vi "test_orientation_tester.vi"() -> ()   [LabVIEW 2026]
uses:
  <vilib>/Utility/error.llb/Trim Whitespace One-Sided.vi
panel:
  out "error out 2":errorcluster
  out "String":string
  out "error out":errorcluster
  in  "Serial Port":refnum<visa-resource-name>="N/A"
  in  "stop":bool
  in  "Tab Control":enum32{"Integrated Circuit Testing"}(tab)
  out "Orientation OK":bool
  out "Detected IC":string
  out "Current":dbl(graph)
  in  "IC Select":u16(ring) items=["7408", "7432", "7404"]
  out "D1":bool
  out "D2":bool
  out "D3":bool
  out "D4":bool
  out "D5":bool
  out "D6":bool
  out "D8":bool
  out "D9":bool
  out "D10":bool
  out "D11":bool
  out "D12":bool
  out "D13":bool
  in  "Start Test":bool
  out "Tests Ran":dbl
  out "PASS":bool
  out "FAIL":bool
  out "Passed":dbl
  out "Failed":dbl
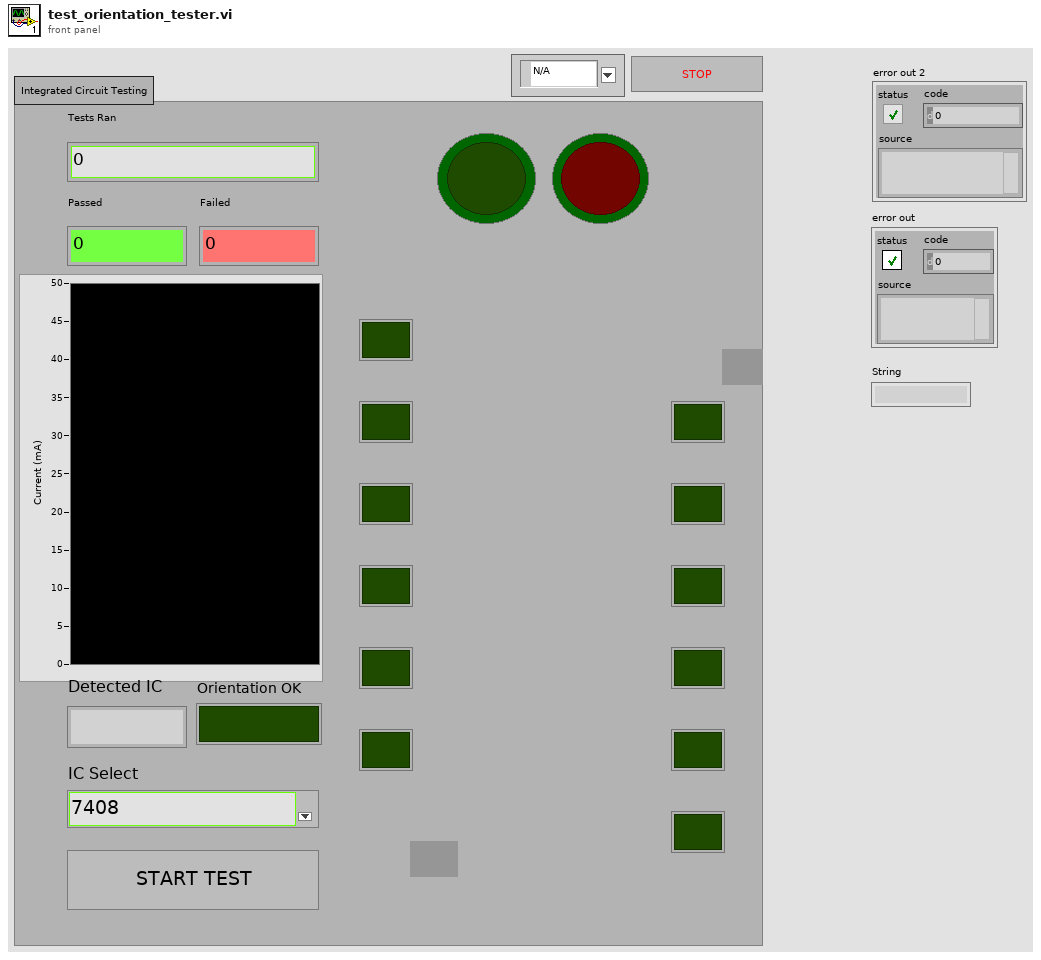
[diagram p1: front panel]
types:
  T1 = enum16{"Standard", "Buffered", "CRLF", "Immediate"}
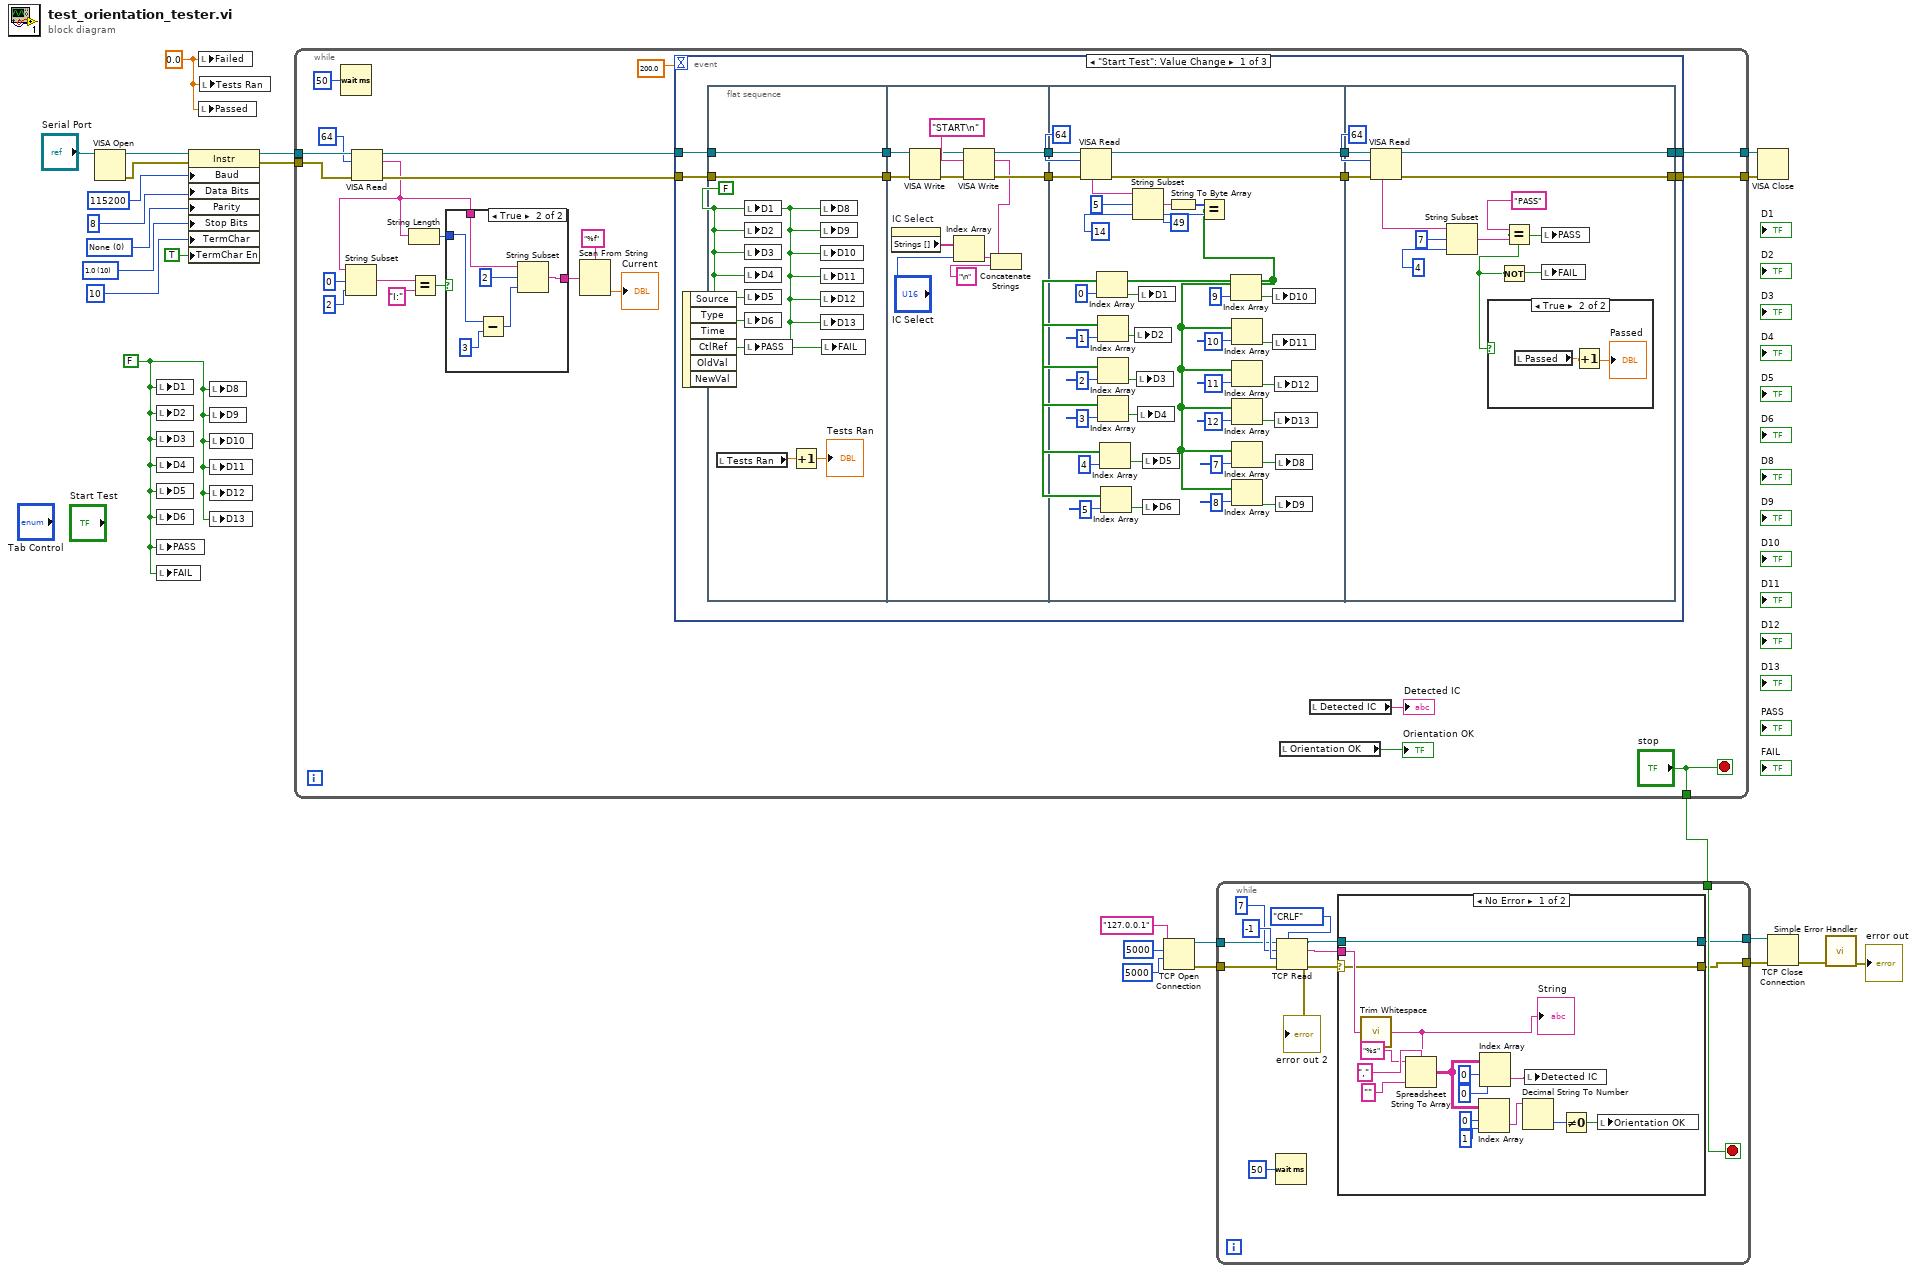
[diagram p0: block diagram]
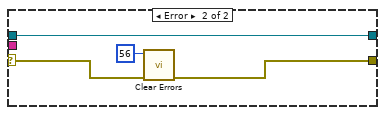
[diagram p2: hidden frame]
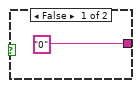
[diagram p3: hidden frame]
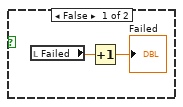
[diagram p4: hidden frame]
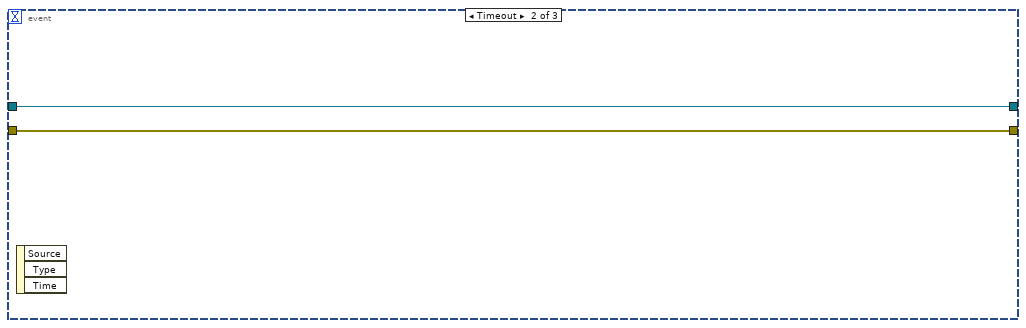
[diagram p5: hidden frame]
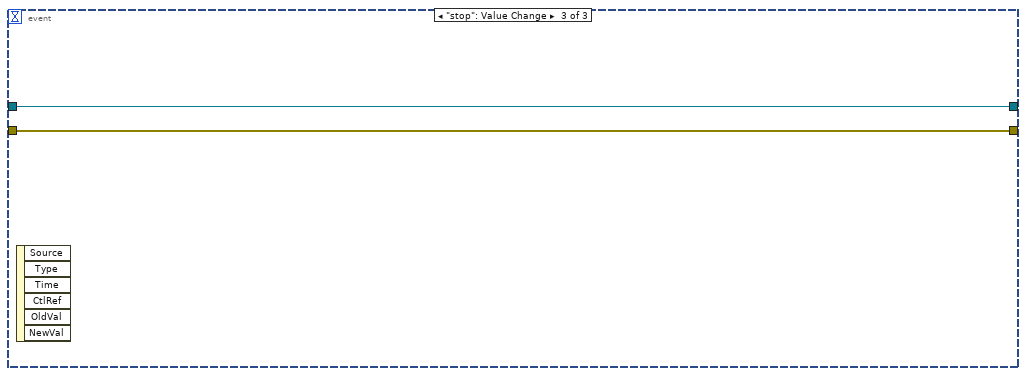
[diagram p6: hidden frame]
diagram:
  w8 = 0.0 ("Failed")
  w12 = FALSE ("D1")
  w17 = u16 10 items=["1.0"=10, "1.5"=15, "2.0"=20] ("Serial Settings:Stop Bits")
  w18 = u16 0 items=["None", "Odd", "Even", "Mark", "Space"] ("Serial Settings:Parity")
  n1 = VISA Open(VISA resource name="Serial Port") -> (VISA resource name=w24:refnum<visa-resource-name>, error out=w22:errorcluster)  [unwired: 4 in]
  n2 = local write "D1"(w12) -> ()
  n3 = local write "D2"(w12) -> ()
  n4 = local write "D3"(w12) -> ()
  n5 = local write "D4"(w12) -> ()
  n6 = local write "D5"(w12) -> ()
  n7 = local write "D6"(w12) -> ()
  n8 = local write "PASS"(w12) -> ()
  n9 = local write "FAIL"(w12) -> ()
  n10 = property class="Instr"(reference=w24, error in=w22, "Baud"=u32 115200 ("Serial Settings:Baud Rate"), "Data Bits"=u16 8 ("Serial Settings:Data Bits"), "Parity"=w18, "Stop Bits"=w17, "TermChar"=u8 10 ("Message Based Settings:Termination Character"), "TermChar En"=TRUE ("Message Based Settings:Termination Character Enable")) -> (reference out=w23:refnum<visa-resource-name>, error out=w21:errorcluster)
  n11 = local write "Failed"(w8) -> ()
  n12 = local write "Passed"(w8) -> ()
  n13 = local write "Tests Ran"(w8) -> ()
  n14 = local write "D8"(w12) -> ()
  n15 = local write "D9"(w12) -> ()
  n16 = local write "D10"(w12) -> ()
  n17 = local write "D11"(w12) -> ()
  n18 = local write "D12"(w12) -> ()
  n19 = local write "D13"(w12) -> ()
  n20 = while {
    tunnel: w23 -> [w47]
    tunnel: w21 -> [w45]
    tunnel: [w42] -> w14
    tunnel: [w41] -> w13
    tunnel: ["stop"] -> w6
    stop <- "stop" stop-if-true
    n21 = Wait (ms)(milliseconds to wait=u32 50) -> ()  [unwired: 1 out]
    n22 = VISA Read(VISA resource name=w47, byte count=u32 64, error in (no error)=w45) -> (VISA resource name out=w44:refnum<visa-resource-name>, read buffer=w35:string, error out=w43:errorcluster)  [unwired: 1 out]
    n23 = String Subset(string=w35, offset (0)=0, length (rest)=2 ("length (rest)")) -> (substring=w34:string)
    n24 = String Length(string=w35) -> (length=w36:i32)
    n25 = Equal?(x=w34, y="I:") -> (x = y?=w33:bool)
    n26 = case shown="True" w33 {
      tunnel: w36 -> [_ w53]
      tunnel: ["0" w50] -> w31
      tunnel: w35 -> [_ w49]
      frame False {
      }
      frame True {
        n27 = Subtract(x=w53, y=3) -> (x-y=w51:i32)
        n28 = String Subset(string=w49, offset (0)=2, length (rest)=w51) -> (substring=w50:string)
      }
    }
    n29 = Scan From String(format string="%f", input string=w31) -> (output 1=→"Current":dbl)  [unwired: 3 in, 3 out]
    n30 = event shown="[0] \"Start Test\": Value Change" {
      selector: _ -> [_ _ _]
      dyn-events: _ -> [_ _ _]
      timeout: 200.0 -> [_ _ _]
      tunnel: w44 -> [w63 w135 w137]
      tunnel: w43 -> [w61 w134 w136]
      tunnel: [w60 w135 w137] -> w42
      tunnel: [w59 w134 w136] -> w41
      event "Start Test": Value Change {
        n31 = event-data() -> ()  [unwired: 1 in, 6 out]
        n32 = flat-sequence {
          tunnel: [w69] -> w64
          tunnel: w63 -> [w69]
          tunnel: [w68] -> w62
          tunnel: w61 -> [w68]
          tunnel: w64 -> [w78]
          tunnel: w62 -> [w76]
          tunnel: [w81] -> w58
          tunnel: [w80] -> w57
          tunnel: w58 -> [w116]
          tunnel: w57 -> [w117]
          tunnel: [w115] -> w56
          tunnel: [w114] -> w55
          tunnel: [w126] -> w59
          tunnel: [w127] -> w60
          tunnel: w56 -> [w129]
          tunnel: w55 -> [w128]
          frame #0 {
            w67 = FALSE ("D1")
            n33 = local read "Tests Ran"() -> (w66:dbl)
            n34 = local write "D1"(w67) -> ()
            n35 = local write "D2"(w67) -> ()
            n36 = local write "D3"(w67) -> ()
            n37 = local write "D4"(w67) -> ()
            n38 = local write "D5"(w67) -> ()
            n39 = local write "D6"(w67) -> ()
            n40 = local write "PASS"(w67) -> ()
            n41 = Increment(x=w66) -> (x+1=→"Tests Ran":dbl)
            n42 = local write "D8"(w67) -> ()
            n43 = local write "D9"(w67) -> ()
            n44 = local write "D10"(w67) -> ()
            n45 = local write "D11"(w67) -> ()
            n46 = local write "D12"(w67) -> ()
            n47 = local write "D13"(w67) -> ()
            n48 = local write "FAIL"(w67) -> ()
          }
          frame #1 {
            n49 = property on="IC Select" class="Ring (strict)"() -> ("Strings []"=w74:string[])  [unwired: 2 in, 2 out]
            n50 = Index Array(array=w74, index="IC Select") -> (element=w72:string)
            n51 = Concatenate Strings(w72, "\n" ("string")) -> (w70:string)
            n52 = VISA Write(VISA resource name=w78, write buffer=w70, error in (no error)=w76) -> (VISA resource name out=w77:refnum<visa-resource-name>, error out=w75:errorcluster)  [unwired: 1 out]
            n53 = VISA Write(VISA resource name=w77, write buffer="START\n", error in (no error)=w75) -> (VISA resource name out=w81:refnum<visa-resource-name>, error out=w80:errorcluster)  [unwired: 1 out]
          }
          frame #2 {
            n54 = VISA Read(VISA resource name=w116, byte count=u32 64, error in (no error)=w117) -> (VISA resource name out=w115:refnum<visa-resource-name>, read buffer=w108:string, error out=w114:errorcluster)  [unwired: 1 out]
            n55 = String Subset(string=w108, offset (0)=5, length (rest)=14 ("length (rest)")) -> (substring=w112:string)
            n56 = String To Byte Array(string=w112) -> (unsigned byte array=w111:u8[])
            n57 = Equal?(x=w111, y=u8 49) -> (x = y?=w83:bool[])
            n58 = Index Array(array=w83, index=0) -> (element=w107:bool)
            n59 = Index Array(array=w83, index=1) -> (element=w103:bool)
            n60 = Index Array(array=w83, index=2) -> (element=w102:bool)
            n61 = Index Array(array=w83, index=3) -> (element=w105:bool)
            n62 = Index Array(array=w83, index=4) -> (element=w106:bool)
            n63 = Index Array(array=w83, index=5) -> (element=w104:bool)
            n64 = local write "D2"(w103) -> ()
            n65 = local write "D3"(w102) -> ()
            n66 = local write "D4"(w105) -> ()
            n67 = local write "D1"(w107) -> ()
            n68 = local write "D5"(w106) -> ()
            n69 = local write "D6"(w104) -> ()
            n70 = Index Array(array=w83, index=9) -> (element=w93:bool)
            n71 = Index Array(array=w83, index=10) -> (element=w92:bool)
            n72 = Index Array(array=w83, index=11) -> (element=w91:bool)
            n73 = Index Array(array=w83, index=12) -> (element=w90:bool)
            n74 = Index Array(array=w83, index=7) -> (element=w95:bool)
            n75 = Index Array(array=w83, index=8) -> (element=w94:bool)
            n76 = local write "D10"(w93) -> ()
            n77 = local write "D11"(w92) -> ()
            n78 = local write "D12"(w91) -> ()
            n79 = local write "D13"(w90) -> ()
            n80 = local write "D8"(w95) -> ()
            n81 = local write "D9"(w94) -> ()
          }
          frame #3 {
            n82 = VISA Read(VISA resource name=w129, byte count=u32 64, error in (no error)=w128) -> (VISA resource name out=w127:refnum<visa-resource-name>, read buffer=w122:string, error out=w126:errorcluster)  [unwired: 1 out]
            n83 = String Subset(string=w122, offset (0)=7, length (rest)=4 ("length (rest)")) -> (substring=w118:string)
            n84 = Equal?(x="PASS", y=w118) -> (x = y?=w119:bool)
            n85 = case shown="True" w119 {
              frame False {
                n86 = local read "Failed"() -> (w130:dbl)
                n87 = Increment(x=w130) -> (x+1=→"Failed":dbl)
              }
              frame True {
                n88 = local read "Passed"() -> (w132:dbl)
                n89 = Increment(x=w132) -> (x+1=→"Passed":dbl)
              }
            }
            n90 = Not(x=w119) -> (.not. x?=w121:bool)
            n91 = local write "PASS"(w119) -> ()
            n92 = local write "FAIL"(w121) -> ()
          }
        }
      }
      event Timeout {
        n93 = event-data() -> ()  [unwired: 1 in, 3 out]
      }
      event "stop": Value Change {
        n94 = event-data() -> ()  [unwired: 1 in, 6 out]
      }
    }
    n95 = local read "Orientation OK"() -> (→"Orientation OK":bool)
    n96 = local read "Detected IC"() -> (→"Detected IC":string)
  }
  n97 = TCP Open Connection(address="127.0.0.1", remote port or service name=u16 5000, timeout ms (60000)=5000) -> (connection ID=w7:refnum<k5>, error out=w4:errorcluster)  [unwired: 2 in]
  n98 = while {
    tunnel: w7 -> [w146]
    tunnel: w6 -> [w145]
    tunnel: [w143] -> w5
    tunnel: w4 -> [w144]
    tunnel: [w140] -> w2
    stop <- w145 stop-if-true
    n99 = Wait (ms)(milliseconds to wait=u32 50) -> ()  [unwired: 1 out]
    n100 = TCP Read(connection ID=w146, bytes to read=7, error in (no error)=w144, 7:T1."CRLF" ("mode (standard)"), 9:-1 ("timeout ms (25000)")) -> (connection ID out=w142:refnum<k5>, data out=w141:string, error out=w138:errorcluster)
    "error out 2" <- w138
    n101 = case shown="No Error" w138 {
      selector: w138 -> [w153 w168]
      tunnel: [w154 w169] -> w143
      tunnel: w142 -> [w154 w169]
      tunnel: w141 -> [w155 _]
      tunnel: [w153 w167] -> w140
      frame No Error {
        n102 = call <vilib>:"Trim Whitespace.vi"("string"=w155) -> ("trimmed string"=w150:string)  [unwired: 1 in]
        "String" <- w150
        n103 = Spreadsheet String To Array(delimiter (Tab)=",", format string="%s", spreadsheet string=w150, array type (2D Dbl)="") -> (array=w165:string[][])
        n104 = Index Array(array=w165, index (row)=0, index (col)=1 ("disabled index (col)")) -> (element=w163:string)
        n105 = Index Array(array=w165, index (row)=0, index (col)=0 ("disabled index (col)")) -> (element=w151:string)
        n106 = Decimal String To Number(string=w163) -> (number=w164:i32)  [unwired: 2 in, 1 out]
        n107 = local write "Detected IC"(w151) -> ()
        n108 = Not Equal To 0?(x=w164) -> (x != 0?=w152:bool)
        n109 = local write "Orientation OK"(w152) -> ()
      }
      frame Error {
        n110 = call <vilib>:"Clear Errors.vi"("error in (no error)"=w168, "specific error code to clear (0: all)"=56) -> ("error out"=w167:errorcluster)  [unwired: 4 in, 1 out]
      }
    }
  }
  n111 = VISA Close(VISA resource name=w14, error in (no error)=w13) -> ()  [unwired: 1 out]
  n112 = TCP Close Connection(connection ID=w5, error in (no error)=w2) -> (error out=w3:errorcluster)  [unwired: 1 in, 1 out]
  n113 = call <vilib>:"Simple Error Handler.vi"("error in (no error)"=w3) -> ("error out"=→"error out":errorcluster)  [unwired: 4 in, 4 out]
